vi "_analyzePortNum_EEPROM_vna_wmg.vi"(0 "cmd_input":string[][](array[string])=[["#0 read #A1 #00 #128", "#0 read #A1 #80 #128", "#0 write #A0 #7F V#01", "#0 read #A1 #80 #128", "#0 write #A0 #7F V#02", "#0 write #A0 #7B K#10 Z#004", "#0 read #A1 #80 #128", "#0 write #A0 #7F V#03", "#0 read #A1 #80 #128", "#0 write #A0 #7F V#00"], ["#1 read #A1 #00 #128", "#1 read #A1 #80 #128", "#1 write #A0 #7F V#01", "#1 read #A1 #80 #128", "#1 write #A0 #7F V#02", "", "", "", "", ""]]) -> (1 "数组C":string[](array[string]), 2 "portNum":i32)   [LabVIEW 2011]
panel:
  out "数组":string[](array[string])
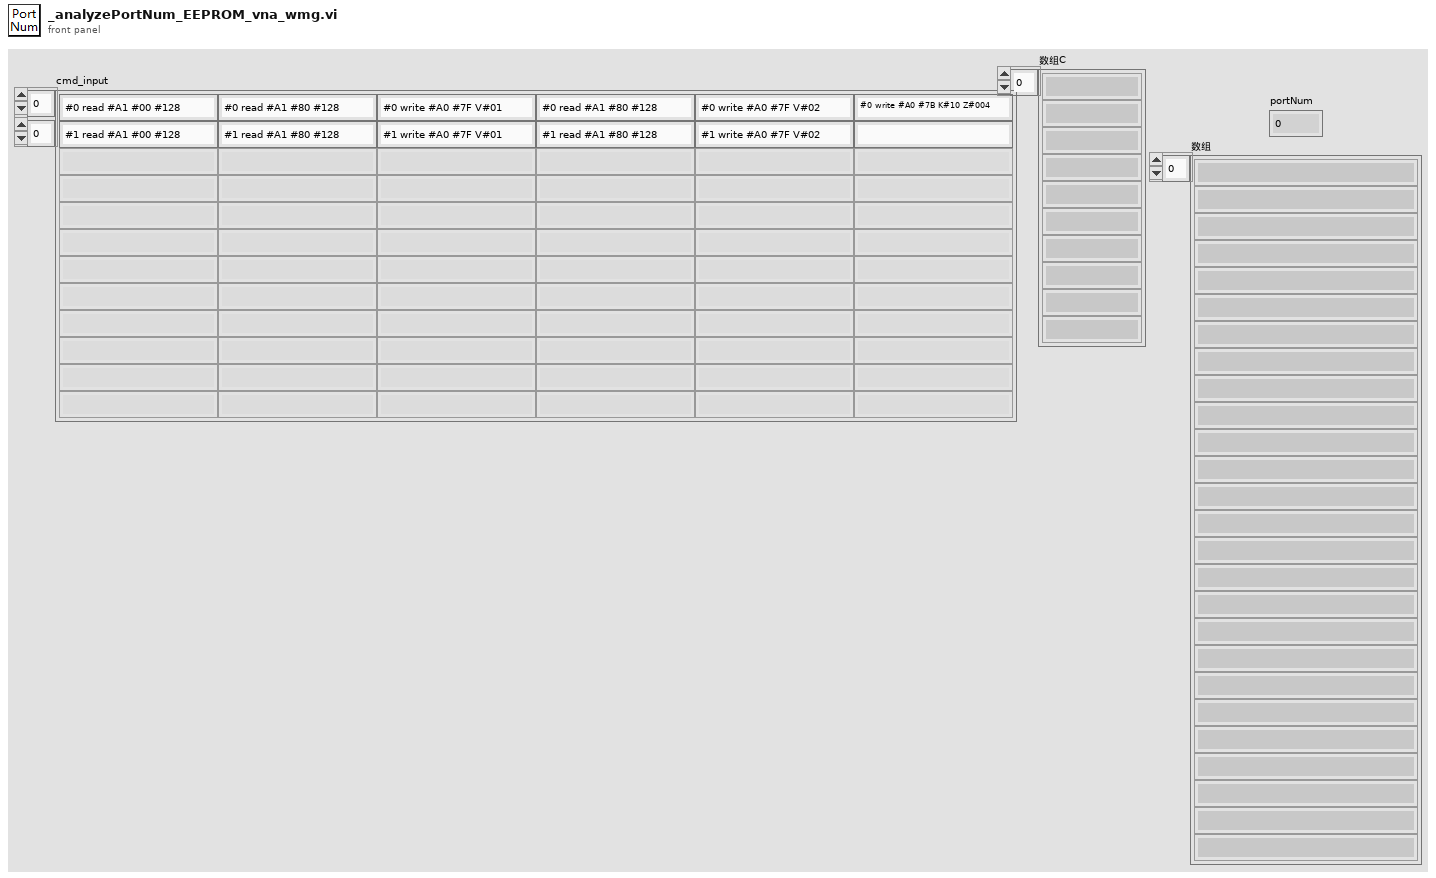
[diagram p1: front panel]
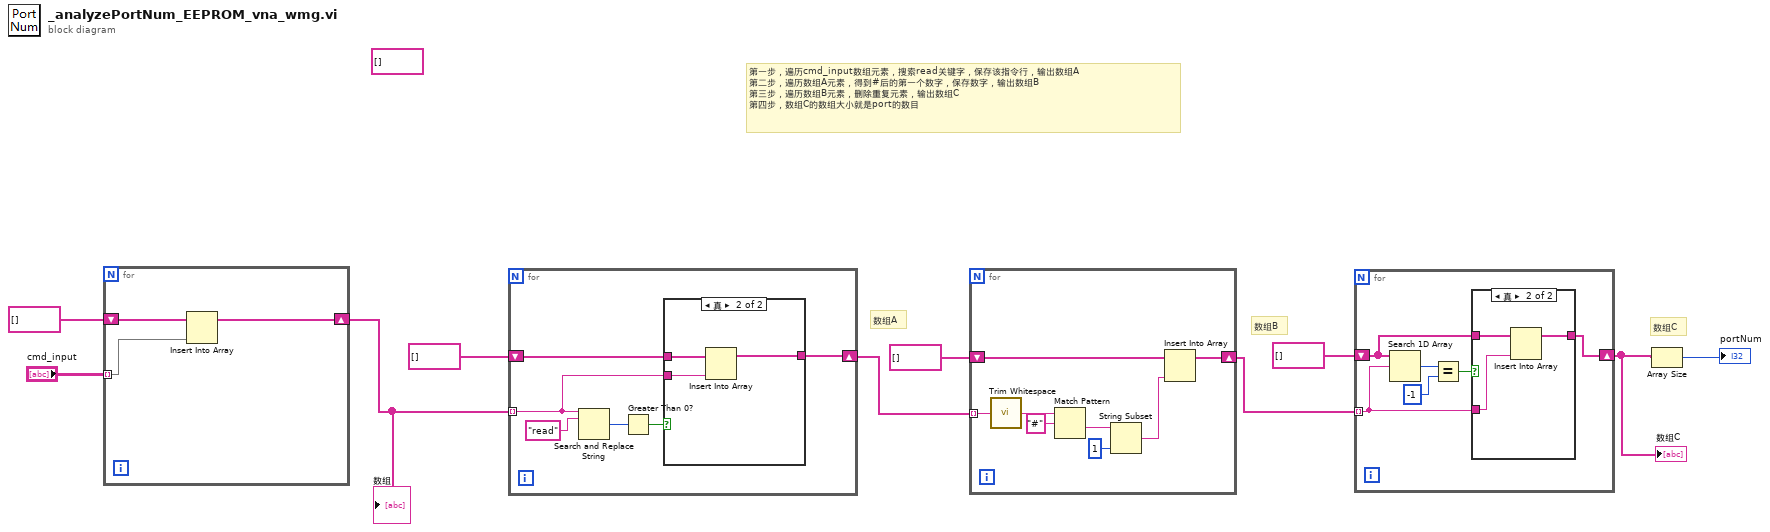
[diagram p0: block diagram]
diagram:
  (unwired) string[] []
  # "数组C"
  # "数组B"
  # "数组A"
  # "第一步，遍历cmd_input数组元素，搜索read关键字，保存该指令行，输出数组A\n第二步，遍历数组A元素，得到#后的第一个数字，保存数字，输出数组B\n第三步，遍历数组B元素，删除重复元素，输出数组C\n第四步，数组C的数组大小就是port的数目"
  n1 = for {
    tunnel: "cmd_input" -> [w12] mode=indexing
    shift-right: [w11] -> w1
    shift-left: string[] [] -> [w13]
    n2 = Insert Into Array(array=w13, new element=w12) -> (w11:string[])  [unwired: 1 in]
  }
  "数组" <- w1
  n3 = for {
    tunnel: w1 -> [w14] mode=indexing
    shift-right: [w15] -> w9
    shift-left: string[] [] -> [w16]
    n4 = Search and Replace String(input string=w14, search string="read" ("搜索字符串")) -> (number of replacements=w18:i32)  [unwired: 6 in, 3 out]
    n5 = Greater Than 0?(x=w18) -> (x > 0?=w17:bool)
    n6 = case shown="真" w17 {
      tunnel: w16 -> [w20 w23]
      tunnel: [w20 w22] -> w15
      tunnel: w14 -> [_ w21]
      frame False {
      }
      frame True {
        n7 = Insert Into Array(array=w23, new element=w21) -> (w22:string[])  [unwired: 1 in]
      }
    }
  }
  n8 = for {
    tunnel: w9 -> [w31] mode=indexing
    shift-right: [w24] -> w7
    shift-left: string[] [] -> [w26]
    n9 = call <vilib>:"Trim Whitespace.vi"("string"=w31) -> ("trimmed string"=w30:string)  [unwired: 1 in]
    n10 = Match Pattern(string=w30, regular expression="#" ("正则表达式")) -> (after substring=w28:string)  [unwired: 1 in, 3 out]
    n11 = String Subset(string=w28, length (rest)=1 ("长度（剩余）")) -> (substring=w25:string)  [unwired: 1 in]
    n12 = Insert Into Array(array=w26, new element=w25) -> (w24:string[])  [unwired: 1 in]
  }
  n13 = for {
    tunnel: w7 -> [w34] mode=indexing
    shift-right: [w32] -> w5
    shift-left: string[] [] -> [w33]
    n14 = Search 1D Array(1D array=w33, element=w34) -> (index of element=w37:i32)  [unwired: 1 in]
    n15 = Equal?(x=w37, y=-1) -> (x = y?=w35:bool)
    n16 = case shown="真" w35 {
      tunnel: w34 -> [_ w40]
      tunnel: w33 -> [w38 w41]
      tunnel: [w38 w39] -> w32
      frame False {
      }
      frame True {
        n17 = Insert Into Array(array=w41, new element=w40) -> (w39:string[])  [unwired: 1 in]
      }
    }
  }
  "数组C" <- w5
  n18 = Array Size(array=w5) -> (size(s)=→"portNum":i32)
